vi "Client Init.vi"(6 "local port (0)":u16, 8 "error in":errorcluster, 9 "remote port (54444)":u16=54444, 10 "server IP address":string, 11 "tag list":T4[](array[typedef])) -> (0 "error out":errorcluster, 3 "connection ID":T1)   [LabVIEW 2010, in "NI_CCC.lvlib"]
doc: "Establishes a client connection with a CVT Client Communication (CCC) server."
uses:
  NI_CCC.lvlib
  Tag Configuration.ctl
  <vilib>/NI/Current Value Table/Type Defs/Data Types.ctl
  Tag Direction.ctl
  Connection ID.ctl
  <vilib>/NI/STM/TCP/TCP Connection Info.ctl
  <vilib>/NI/STM/SubVIs/MetaDataElement.ctl
  <vilib>/NI/STM/TCP/TCP Read Options.ctl
  Read Error.vi
  Initialize Address_Index Lists.vi
  <vilib>/NI/Current Value Table/Get Index and Type.vi
  <vilib>/NI/Current Value Table/Group Tags.vi
  <vilib>/NI/STM/TCP/Read Meta Data (TCP Clst).vi
  FG Client Configurations.vi
  <vilib>/NI/STM/TCP/Write Message (TCP).vi
  <vilib>/NI/Current Value Table/FGVs/Tag Memory.vi
  <vilib>/NI/Current Value Table/FGVs/Group Memory.vi
  <vilib>/NI/Current Value Table/Form Single Group.vi
  <vilib>/NI/STM/TCP/Read Message (TCP).vi
  <vilib>/NI/STM/NI STM.lvlib
  <vilib>/NI/Current Value Table/Current Value Table.lvlib
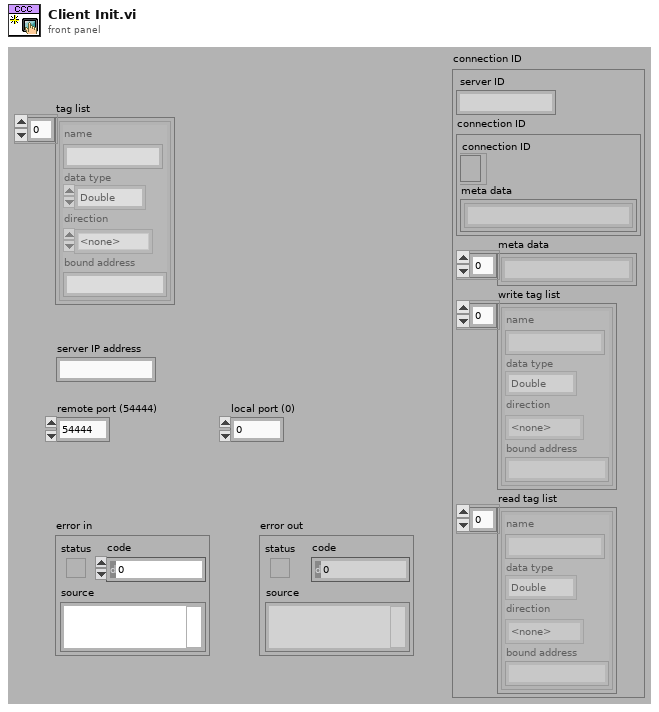
[diagram p1: front panel]
types:
  T1 = typedef "NI_CCC.lvlib/Connection ID.ctl" = cluster{"server ID":string, "connection ID":T2, "meta data":T3[], "write tag list":T4[], "read tag list":T4[]}
  T2 = typedef "NI STM.lvlib/TCP Connection Info.ctl" = cluster{"connection ID":refnum<k5>, "meta data":T3[]}
  T3 = typedef "NI STM.lvlib/MetaDataElement.ctl" = string
  T4 = typedef "NI_CCC.lvlib/Tag Configuration.ctl" = cluster{"name":string, "data type":T5, "direction":T6, "bound address":string}
  T5 = typedef "Current Value Table.lvlib/Data Types.ctl" = enum16{"Double", "Single", "I64", "I32", "I16", "I8", "U64", "U32", "U16", "U8", "String", "Boolean", "Array of U8", "Array of U16", "Array of U32", "Array of U64", "Array of I64", "Array of I32", "Array of I16", "Array of I8", "Array of Double", "Array of Single", "Array of Boolean", "Array of String"}
  T6 = typedef "NI_CCC.lvlib/Tag Direction.ctl" = enum32{"<none>", "Read", "Write"}
  T7 = typedef "NI STM.lvlib/TCP Read Options.ctl" = cluster{"ignore timeout error":bool, "timeout ms (1000)":i32}
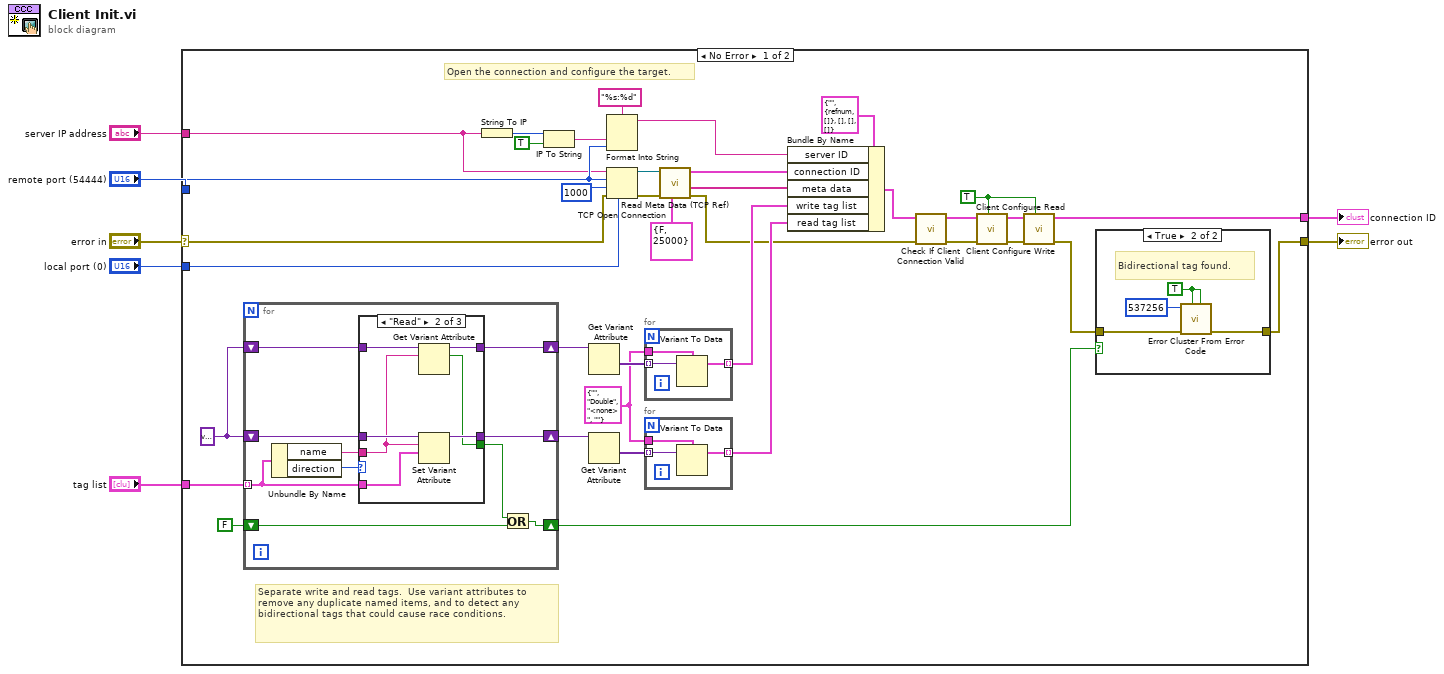
[diagram p0: block diagram]
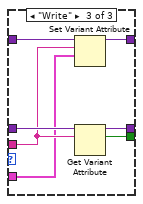
[diagram p4: hidden frame]
diagram:
  n1 = case shown="No Error" "error in" {
    selector: "error in" -> [w44 w82]
    tunnel: "tag list" -> [w13 _]
    tunnel: [w9 w82] -> w6
    tunnel: [w19 _] -> w5
    tunnel: "remote port (54444)" -> [w28 _]
    tunnel: "server IP address" -> [w23 _]
    tunnel: "local port (0)" -> [w29 _]
    frame No Error {
      w18 = TRUE ("force configure? (F)")
      w31 = T4 {"name"="", "data type"=enum."Double", "direction"=enum."<none>", "bound address"=""} ("tag configuration")
      w12 = variant ("tag list")
      # "Open the connection and configure the target."
      # "Separate write and read tags.  Use variant attributes to remove any duplicate named items, and to detect any bidirectional tags that could cause race conditions."
      n2 = for {
        tunnel: w13 -> [w61] mode=indexing
        shift-right: [w64] -> w35
        shift-left: w12 -> [w65]
        shift-right: [w62] -> w36
        shift-left: w12 -> [w63]
        shift-right: [w57] -> w10
        shift-left: FALSE -> [w56]
        n3 = Unbundle By Name(w61) -> ("name"=w59:string, "direction"=w60:T6)
        n4 = case shown="\"Read\"" w60 {
          tunnel: w65 -> [w67 w71 w81]
          tunnel: [w67 w70 w80] -> w64
          tunnel: w63 -> [w66 w72 w79]
          tunnel: [w66 w73 w78] -> w62
          tunnel: w61 -> [_ w74 w76]
          tunnel: w59 -> [_ w69 w77]
          tunnel: [_ w68 w75] -> w58
          frame "<none>" {
          }
          frame "Read" {
            n5 = Get Variant Attribute(Variant=w71, name=w69) -> (duplicate Variant=w70:variant, found=w68:bool)  [unwired: 2 in, 2 out]
            n6 = Set Variant Attribute(Variant=w72, name=w69, value=w74) -> (Variant out=w73:variant)  [unwired: 1 in, 2 out]
          }
          frame "Write" {
            n7 = Set Variant Attribute(Variant=w81, name=w77, value=w76) -> (Variant out=w80:variant)  [unwired: 1 in, 2 out]
            n8 = Get Variant Attribute(Variant=w79, name=w77) -> (duplicate Variant=w78:variant, found=w75:bool)  [unwired: 2 in, 2 out]
          }
        }
        n9 = Or(x=w58, y=w56) -> (x .or. y?=w57:bool)
      }
      n10 = String To IP(1:w23) -> (0:w24:u32)
      n11 = IP To String(1:TRUE ("dot notation? (F)"), 2:w24) -> (0:w22:string)
      n12 = Get Variant Attribute(Variant=w35) -> (values=w34:variant[])  [unwired: 3 in, 3 out]
      n13 = Get Variant Attribute(Variant=w36) -> (values=w32:variant[])  [unwired: 3 in, 3 out]
      n14 = Format Into String(format string="%s:%d", w22, w28) -> (resulting string=w26:string)  [unwired: 2 in, 1 out]
      n15 = TCP Open Connection(address=w23, remote port or service name=w28, timeout ms (60000)=1000, local port=w29, error in (no error)=w44) -> (connection ID=w43:refnum<k5>, error out=w42:errorcluster)
      n16 = for {
        tunnel: w34 -> [w55] mode=indexing
        tunnel: w31 -> [w54]
        tunnel: [w53] -> w33 mode=indexing
        n17 = Variant To Data(Variant=w55, type=w54) -> (data=w53:T4)  [unwired: 1 in, 1 out]
      }
      n18 = for {
        tunnel: w32 -> [w52] mode=indexing
        tunnel: w31 -> [w51]
        tunnel: [w50] -> w30 mode=indexing
        n19 = Variant To Data(Variant=w52, type=w51) -> (data=w50:T4)  [unwired: 1 in, 1 out]
      }
      n20 = call <vilib>:"Read Meta Data (TCP Ref).vi"("options"=T7 {"ignore timeout error"=FALSE, "timeout ms (1000)"=25000} ("Options"), "error in"=w42, "connection ID"=w43) -> ("error out"=w15:errorcluster, "meta data"=w40:T3[], "connection info out"=w41:T2)  [unwired: 6 in]
      n21 = Bundle By Name(cluster=T1 {"server ID"="", "connection ID"={"connection ID"=refnum, "meta data"=[]}, "meta data"=[], "write tag list"=[], "read tag list"=[]} ("CCC Connection ID"), "server ID"=w26, "connection ID"=w41, "meta data"=w40, "write tag list"=w33, "read tag list"=w30) -> (w17:T1)
      n22 = call "Check If Client Connection Valid.vi"("error in"=w15, "connection ID in"=w17) -> ("error out"=w14:errorcluster, "connection ID out"=w16:T1)  [unwired: 7 in, 1 out]
      n23 = call "Client Configure Read.vi"("force configure? (F)"=w18, "error in"=w14, "connection ID in"=w16) -> ("error out"=w20:errorcluster, "connection ID out"=w21:T1)  [unwired: 5 in, 2 out]
      n24 = call "Client Configure Write.vi"("force configure? (F)"=w18, "error in"=w20, "connection ID in"=w21) -> ("error out"=w8:errorcluster, "connection ID out"=w19:T1)  [unwired: 5 in, 2 out]
      n25 = case shown="True" w10 {
        tunnel: w8 -> [w45 w48]
        tunnel: [w45 w46] -> w9
        frame False {
        }
        frame True {
          w47 = TRUE ("show call chain? (False)")
          # "Bidirectional tag found."
          n26 = call <vilib>:"Error Cluster From Error Code.vi"("is warning? (False)"=w47, "show call chain? (False)"=w47, "error in (no error)"=w48, "error code (0)"=537256) -> ("error out"=w46:errorcluster)  [unwired: 5 out]
        }
      }
    }
    frame Error {
    }
  }
  "connection ID" <- w5
  "error out" <- w6
